vi "Blend colors with alpha.vi"(9 "Top alpha":dbl=1.0 min=0.0 max=1.0, 10 "Bottom color":u32(colorbox), 11 "Top color":u32(colorbox)) -> (2 "Result alpha":dbl min=0.0 max=1.0, 3 "Result color":u32(colorbox))   [LabVIEW 2023]
panel:
  in  "Bottom alpha":dbl=1.0 min=0.0 max=1.0
  # "0 = Transparent\n1 = Opaque"
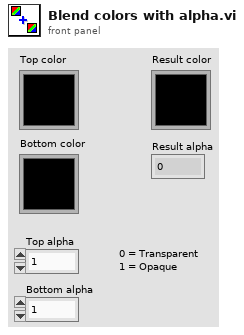
[diagram p1: front panel]
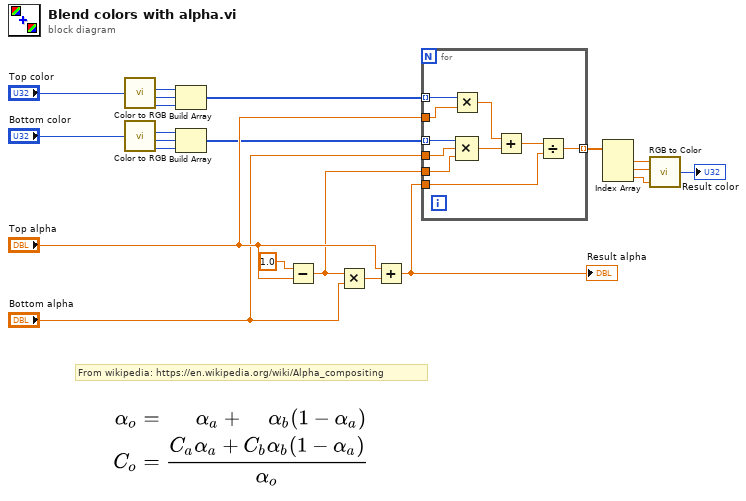
[diagram p0: block diagram]
diagram:
  # "From wikipedia: https://en.wikipedia.org/wiki/Alpha_compositing"
  n1 = call <vilib>:"Color to RGB.vi"("Color"="Top color") -> ("R"=w18:u8, "G"=w17:u8, "B"=w16:u8)  [unwired: 1 out]
  n2 = call <vilib>:"Color to RGB.vi"("Color"="Bottom color") -> ("R"=w13:u8, "G"=w14:u8, "B"=w15:u8)  [unwired: 1 out]
  n3 = Build Array(w18, w17, w16) -> (w9:u8[])
  n4 = Build Array(w13, w14, w15) -> (w8:u8[])
  n5 = Subtract(x=1.0, y="Top alpha") -> (x-y=w7:dbl)
  n6 = Multiply(x=w7, y="Bottom alpha") -> (x*y=w20:dbl)
  n7 = Add(x="Top alpha", y=w20) -> (x+y=w1:dbl)
  "Result alpha" <- w1
  n8 = for {
    tunnel: w9 -> [w31] mode=indexing
    tunnel: "Top alpha" -> [w24]
    tunnel: "Bottom alpha" -> [w29]
    tunnel: w8 -> [w30] mode=indexing
    tunnel: w7 -> [w28]
    tunnel: [w23] -> w6 mode=indexing
    tunnel: w1 -> [w22]
    n9 = Multiply(x=w31, y=w24) -> (x*y=w26:dbl)
    n10 = Compound Arithmetic op=MULTIPLY(w30, w29, w28) -> (w27:dbl)
    n11 = Add(x=w26, y=w27) -> (x+y=w25:dbl)
    n12 = Divide(x=w25, y=w22) -> (x/y=w23:dbl)
  }
  n13 = Index Array(array=w6) -> (element #1=w5:dbl, element #2=w4:dbl, element #3=w3:dbl)  [unwired: 3 in]
  n14 = call <vilib>:"RGB to Color.vi"("B"=w3, "G"=w4, "R"=w5) -> ("Color"=→"Result color":u32)
